vi "Parameter(FGV).vi"(6 "Parameter Method":T1(ring), 8 "error in":errorcluster, 11 "Parameter In":T2) -> (0 "error out":errorcluster, 3 "Parameter Out":T2)   [LabVIEW 2018]
uses:
  Data Def/Parameter.ctl
  Data Def/Channel Count.ctl
  Data Def/Frequency Setting.ctl
  Data Def/Signal Type Setting.ctl
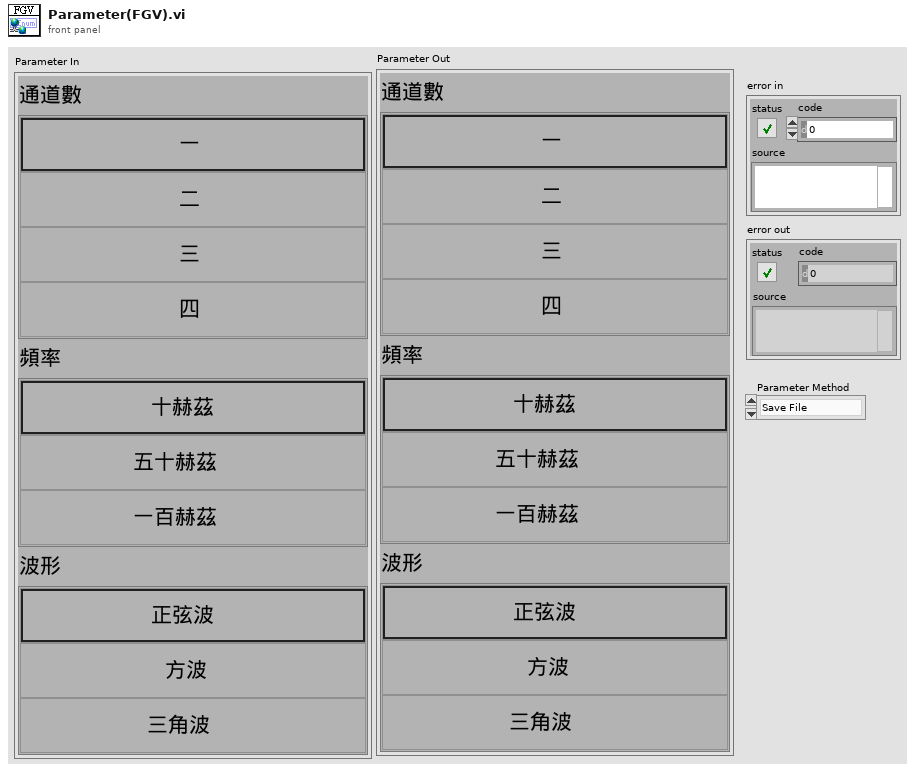
[diagram p1: front panel]
types:
  T1 = enum16{"Save File", "Read File", "Put Frequency", "Put Signal Type", "Put Channel", "Put All", "Get All"}
  T2 = typedef "Parameter.ctl" = cluster{"Channel Count":T3, "Frequency Setting":T4, "Signal Type Setting":T5}
  T3 = typedef "Channel Count.ctl" = enum32{"1", "2", "3", "4"}
  T4 = typedef "Frequency Setting.ctl" = enum32{"10 Hz", "50 Hz", "100 Hz"}
  T5 = typedef "Signal Type Setting.ctl" = enum32{"Sine", "Sqaure", "Triangle"}
  T6 = enum16{"open", "replace", "create", "open or create", "replace or create", "replace or create with confirmation"}
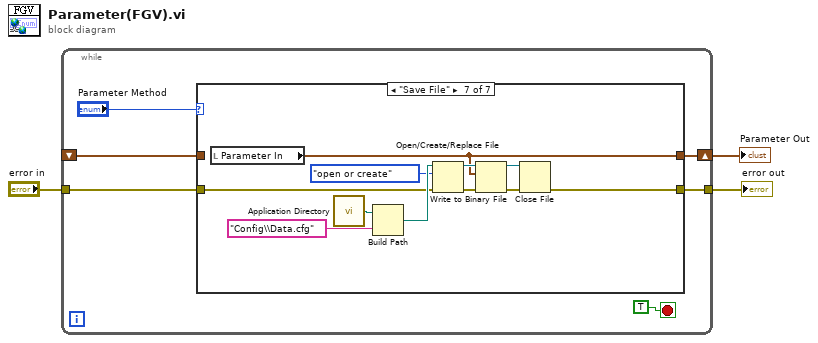
[diagram p0: block diagram]
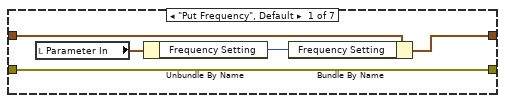
[diagram p2: hidden frame]
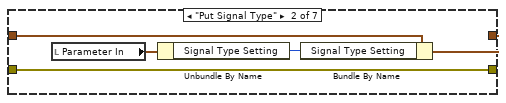
[diagram p3: hidden frame]
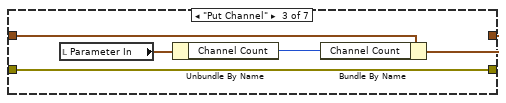
[diagram p4: hidden frame]
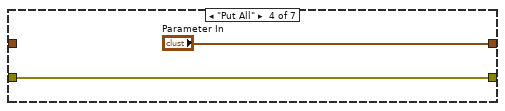
[diagram p5: hidden frame]
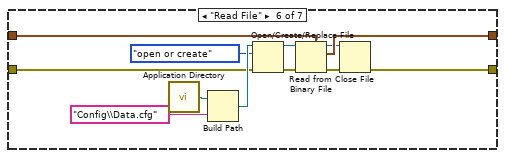
[diagram p7: hidden frame]
diagram:
  n1 = while {
    shift-right: [w7] -> w3
    shift-left: _ -> [w6]
    tunnel: [w5] -> w2
    tunnel: "error in" -> [w4]
    stop <- TRUE stop-if-true
    n2 = case shown="\"Save File\"" "Parameter Method" {
      tunnel: [w11 w16 w22 "Parameter In" w28 w33 w41] -> w7
      tunnel: w6 -> [w14 w17 w23 _ w28 w34 _]
      tunnel: [w10 w15 w20 w25 w27 w30 w42] -> w5
      tunnel: w4 -> [w10 w15 w20 w25 w27 w29 w47]
      frame "Put Frequency", Default {
        n3 = local read "Parameter In"() -> (w13:T2)
        n4 = Unbundle By Name(w13) -> ("Frequency Setting"=w12:T4)
        n5 = Bundle By Name(cluster=w14, "Frequency Setting"=w12) -> (w11:T2)
      }
      frame "Put Signal Type" {
        n6 = local read "Parameter In"() -> (w19:T2)
        n7 = Unbundle By Name(w19) -> ("Signal Type Setting"=w18:T5)
        n8 = Bundle By Name(cluster=w17, "Signal Type Setting"=w18) -> (w16:T2)
      }
      frame "Put Channel" {
        n9 = local read "Parameter In"() -> (w24:T2)
        n10 = Unbundle By Name(w24) -> ("Channel Count"=w21:T3)
        n11 = Bundle By Name(cluster=w23, "Channel Count"=w21) -> (w22:T2)
      }
      frame "Put All" {
      }
      frame "Get All" {
      }
      frame "Read File" {
        n12 = call <vilib>:"Application Directory.vi"() -> ("Application Directory"=w40:path)
        n13 = Build Path(base path=w40, name or relative path="Config\\Data.cfg") -> (appended path=w38:path)
        n14 = Open/Create/Replace File(file path (use dialog)=w38, error in=w29, operation (0:open)=T6."open or create") -> (refnum out=w35:refnum<file>, error out=w36:errorcluster)  [unwired: 3 in, 1 out]
        n15 = Read from Binary File(5:w34, 8:w36, 11:w35) -> (0:w32:errorcluster, 2:w33:T2, 3:w31:refnum<file>)  [unwired: 3 in, 1 out]
        n16 = Close File(refnum=w31, error in=w32) -> (error out=w30:errorcluster)  [unwired: 1 out]
      }
      frame "Save File" {
        n17 = local read "Parameter In"() -> (w41:T2)
        n18 = call <vilib>:"Application Directory.vi"() -> ("Application Directory"=w51:path)
        n19 = Build Path(base path=w51, name or relative path="Config\\Data.cfg") -> (appended path=w49:path)
        n20 = Open/Create/Replace File(file path (use dialog)=w49, error in=w47, operation (0:open)=T6."open or create") -> (refnum out=w43:refnum<file>, error out=w46:errorcluster)  [unwired: 3 in, 1 out]
        n21 = Write to Binary File(file (use dialog)=w43, data=w41, error in=w46) -> (refnum out=w44:refnum<file>, error out=w45:errorcluster)  [unwired: 3 in, 1 out]
        n22 = Close File(refnum=w44, error in=w45) -> (error out=w42:errorcluster)  [unwired: 1 out]
      }
    }
  }
  "error out" <- w2
  "Parameter Out" <- w3
